vi "LowIF_audiojack_exe_beep.vi"() -> ()   [LabVIEW 2015]
doc: "This example demonstrates how to use the Short-time Fourier Transform (STFT Spectrograms) VI to analyze the Time-Frequency spectrogram."
uses:
  <vilib>/sound2/lvsound2.llb/Sampling Mode.ctl
  <vilib>/Analysis/3filter.llb/Filter Passband Type.ctl
  <vilib>/Analysis/2dsp.llb/Complex FFT.vi
  <vilib>/sound2/lvsound2.llb/Sound Input Read (DBL).vi
  <vilib>/Analysis/3filter.llb/Chebyshev Filter (DBL).vi
  <vilib>/Analysis/baseanly.llb/Mean (CDB).vi
  HeartRate_Global.vi
  <vilib>/Analysis/NI_AALPro.lvlib
  <vilib>/Analysis/NI_AALBase.lvlib
  <vilib>/Analysis/NI_AAL_SigProc.lvlib
panel:
  in  "Data path":path=path "test.lvm" caption="Filename"
  in  "Save":bool=TRUE caption="Enable"
  in  "Beep?":bool=TRUE
  out "Heart rate":dbl format="%#.0f"
  out "Respiration rate":dbl format="%#.0f"
  in  "Minimun dB":dbl=-15.0 max=0.0
  in  "Frequency Range":dbl(slide)=3.2 caption="Beats per Min (x60)" min=1.0 step=0.1 scale=0.0..160.0
  out "Frequency":dbl[](graph) caption="I/Q Signal"
  in  "bits per sample":i32=16
  in  "number of channels":i32=2
  in  "sample rate (S/s)":dbl=320.0
  in  "data length":i32=4800
  out "I/Q Signal":dynamicdata(graph)
  in  "number of samples/ch":i32=32
  in  "device ID":u32
  in  "Stop":bool
  # "Low-IF interferometry radar data processing"
  # "Version: 3\nZhengyu Peng\nC. Li Lab\nTexas Tech University\nOct. 2015"
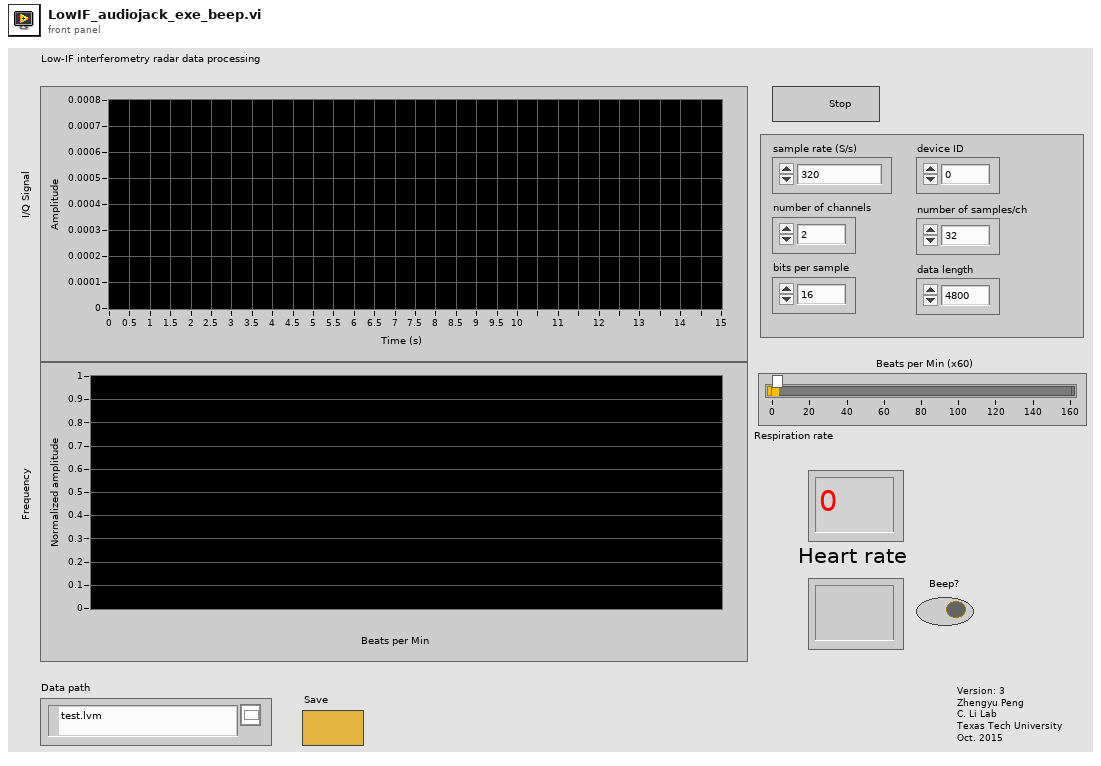
[diagram p1: front panel]
types:
  T1 = typedef "Sampling Mode.ctl" = i32
  T2 = cluster{"sample rate (S/s)":dbl, "number of channels":i32, "bits per sample ":i32}
  T3 = typedef "Sound Input Task ID.ctl" = u32
  T4 = typedef "NI_AALBase.lvlib/Filter Passband Type.ctl" = enum32{"Lowpass", "Highpass", "Bandpass", "Bandstop"}
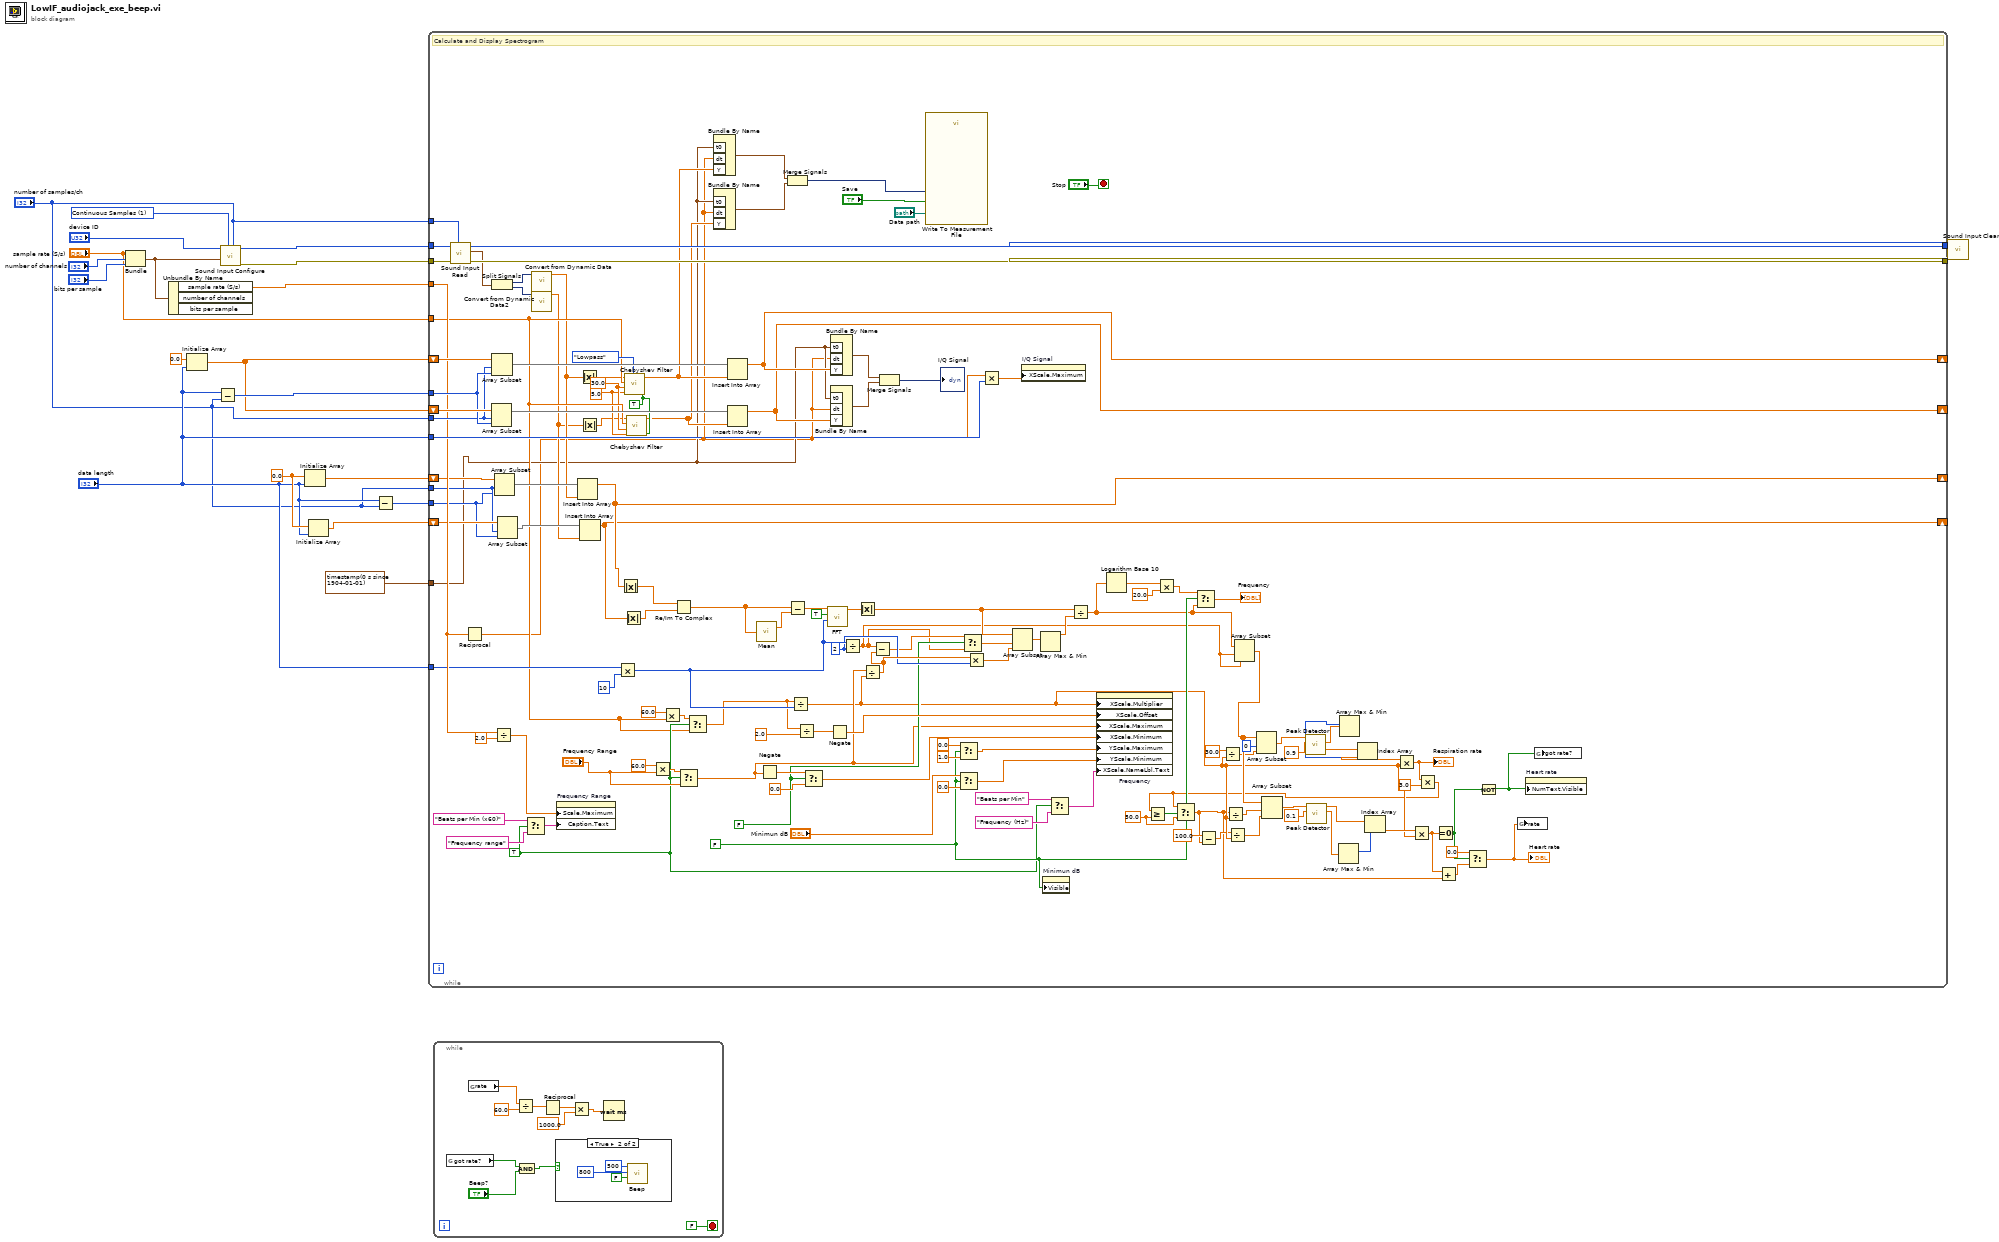
[diagram p0: block diagram]
diagram:
  w4 = T1 1 items=["Finite Samples", "Continuous Samples"] ("sample mode")
  w9 = 0.0 ("element")
  n1 = Bundle("sample rate (S/s)"="sample rate (S/s)", "number of channels"="number of channels", "bits per sample"="bits per sample") -> (w5:T2)  [unwired: 1 in]
  n2 = Unbundle By Name(w5) -> ("sample rate (S/s)"=w13:dbl)  [unwired: 2 out]
  n3 = Initialize Array(0.0 ("element"), "data length") -> (w14:dbl[])
  n4 = Subtract(x="data length", y="number of samples/ch") -> (x-y=w15:i32)
  n5 = call <vilib>:"Sound Input Configure.vi"("number of samples/ch"="number of samples/ch", "sample mode"=w4, "sound format"=w5, "device ID"="device ID") -> ("error out"=w19:errorcluster, "task ID"=w20:T3)  [unwired: 6 in]
  n6 = Initialize Array(w9, "data length") -> (w11:dbl[])
  n7 = Initialize Array(w9, "data length") -> (w8:dbl[])
  n8 = Subtract(x="data length", y="number of samples/ch") -> (x-y=w10:i32)
  n9 = while {
    tunnel: w20 -> [w156]
    tunnel: "number of samples/ch" -> [w155]
    tunnel: w19 -> [w154]
    tunnel: [w153] -> w18
    tunnel: [w152] -> w17
    shift-right: [w137] -> _
    shift-left: w14 -> [w149]
    tunnel: w15 -> [w146]
    shift-right: [w136] -> _
    shift-left: w14 -> [w147]
    tunnel: "number of samples/ch" -> [w143]
    tunnel: w13 -> [w139]
    tunnel: "data length" -> [w141]
    tunnel: "data length" -> [w123]
    tunnel: "sample rate (S/s)" -> [w64]
    shift-right: [w81] -> _
    shift-left: w11 -> [w129]
    tunnel: w10 -> [w125]
    tunnel: "number of samples/ch" -> [w126]
    shift-right: [w79] -> _
    shift-left: w8 -> [w127]
    tunnel: timestamp(0 s since 1904-01-01) ("t0") -> [w28]
    stop <- "Stop" stop-if-true
    w39 = 50.0 ("y")
    w63 = 30.0 ("high cutoff freq: fh")
    w61 = TRUE ("init/cont (init:F)")
    w62 = 5.0 ("high cutoff freq: fh")
    w107 = FALSE ("negative frequency?")
    w97 = FALSE ("dB scale?")
    w84 = TRUE ("scale to beats per min?")
    w110 = 2 ("y")
    # "Calculate and Display Spectrogram"
    n10 = call-poly <vilib>:"Sound Input Read.vi"("number of samples/ch"=w155, "error in (no error)"=w154, "task ID"=w156) -> ("error out"=w152:errorcluster, "data"=w33:waveform(dbl)[], "task ID out"=w153:T3)  [unwired: 6 in]
    n11 = Reciprocal(x=w139) -> (1/x=w27:dbl)
    n12 = Array Subset(array=w147, index=w143, length=w146) -> (w145:dbl[])
    n13 = Split Signals(w33) -> (w151:dynamicdata, w150:dynamicdata)  [unwired: 2 out]
    n14 = Array Subset(array=w149, index=w143, length=w146) -> (w148:dbl[])
    n15 = Divide(x=w139, y=2.0) -> (x/y=w120:dbl)
    n16 = Array Subset(array=w129, index=w126, length=w125) -> (w128:dbl[])
    n17 = Array Subset(array=w127, index=w126, length=w125) -> (w124:dbl[])
    n18 = Select(t="Beats per Min (x60)" ("X Scale.Name Label.Text"), s=w84, f="Frequency range" ("X Scale.Name Label.Text")) -> (s? t:f=w83:string)
    n19 = call "Convert from Dynamic Data"("Dynamic Data Type"=w151) -> ("Array"=w36:dbl[])  [unwired: 3 out]
    n20 = call "Convert from Dynamic Data2"("Dynamic Data Type"=w150) -> ("Array"=w35:dbl[])  [unwired: 3 out]
    n21 = property on="Frequency Range" class="Slide (strict)"("Scale.Maximum"=w120, "Caption.Text"=w83) -> ()  [unwired: 2 in, 2 out]
    n22 = Insert Into Array(array=w128, new element=w36) -> (w81:dbl[])  [unwired: 1 in]
    n23 = Absolute Value(x=w36) -> (abs(x)=w38:dbl[])
    n24 = Absolute Value(x=w35) -> (abs(x)=w37:dbl[])
    n25 = Insert Into Array(array=w124, new element=w35) -> (w79:dbl[])  [unwired: 1 in]
    n26 = Multiply(x=w123, y=10) -> (x*y=w113:i32)
    n27 = Absolute Value(x=w81) -> (abs(x)=w80:dbl[])
    n28 = Absolute Value(x=w79) -> (abs(x)=w78:dbl[])
    n29 = call-poly <vilib>:"Chebyshev Filter.vi"("init/cont (init:F)"=w61, "filter type"=Filter_Passband_Type."Lowpass", "low cutoff freq: fl"=w62, "high cutoff freq: fh"=w63, "sampling freq: fs"=w64, "X"=w38) -> ("Filtered X"=w30:dbl[])  [unwired: 4 in, 1 out]
    n30 = call-poly <vilib>:"Chebyshev Filter.vi"("init/cont (init:F)"=w61, "low cutoff freq: fl"=w62, "high cutoff freq: fh"=w63, "sampling freq: fs"=w64, "X"=w37) -> ("Filtered X"=w29:dbl[])  [unwired: 5 in, 1 out]
    n31 = Multiply(x=60.0, y="Frequency Range") -> (x*y=w89:dbl)
    n32 = Multiply(x=60.0, y=w64) -> (x*y=w92:dbl)
    n33 = Re/Im To Complex(1:w78, 2:w80) -> (0:w82:cdb[])
    n34 = Select(t=w89, s=w84, f="Frequency Range") -> (s? t:f=w88:dbl)
    n35 = Select(t=w92, s=w84, f=w64) -> (s? t:f=w91:dbl)
    n36 = Bundle By Name("t0"=w28, "dt"=w27, "Y"=w30) -> (w26:waveform(dbl))  [unwired: 1 out]
    n37 = Bundle By Name("t0"=w28, "dt"=w27, "Y"=w29) -> (w25:waveform(dbl))  [unwired: 1 out]
    n38 = Insert Into Array(array=w148, new element=w30) -> (w137:dbl[])  [unwired: 1 in]
    n39 = Insert Into Array(array=w145, new element=w29) -> (w136:dbl[])  [unwired: 1 in]
    n40 = call-poly <vilib>:"Mean.vi"("X"=w82) -> ("mean"=w135:cdb)  [unwired: 1 out]
    n41 = Negate(x=w88) -> (-x=w117:dbl)
    n42 = Merge Signals(w26, w25) -> (w24:dynamicdata)
    n43 = Subtract(x=w82, y=w135) -> (x-y=w121:cdb[])
    n44 = Divide(x=w91, y=w113) -> (x/y=w50:dbl)
    n45 = Divide(x=w91, y=2.0) -> (x/y=w131:dbl)
    n46 = Select(t=w117, s=w107, f=0.0) -> (s? t:f=w119:dbl)
    n47 = call-poly <vilib>:"FFT.vi"("FFT size"=w113, "shift?"=TRUE, "X"=w121) -> ("FFT {X}"=w133:cdb[])  [unwired: 7 in, 1 out]
    n48 = Negate(x=w131) -> (-x=w130:dbl)
    n49 = Bundle By Name("t0"=w28, "dt"=w27, "Y"=w137) -> (w144:waveform(dbl))  [unwired: 1 out]
    n50 = Bundle By Name("t0"=w28, "dt"=w27, "Y"=w136) -> (w142:waveform(dbl))  [unwired: 1 out]
    n51 = Divide(x=w113, y=w110) -> (x/y=w47:dbl)
    n52 = Absolute Value(x=w133) -> (abs(x)=w116:dbl[])
    n53 = Divide(x=w88, y=w50) -> (x/y=w111:dbl)
    n54 = Subtract(x=w47, y=w111) -> (x-y=w108:dbl)
    n55 = Merge Signals(w144, w142) -> (→"I/Q Signal":dynamicdata)
    n56 = call "Write To Measurement File"("Signals"=w24, "Enable"="Save", "Filename"="Data path") -> ()  [unwired: 14 in, 3 out]
    n57 = Select(t=0.0, s=w97, f=1.0) -> (s? t:f=w99:dbl)
    n58 = Select(t="Minimun dB", s=w97, f=0.0) -> (s? t:f=w103:dbl)
    n59 = Select(t=w108, s=w107, f=w47) -> (s? t:f=w109:dbl)
    n60 = Multiply(x=w111, y=w110) -> (x*y=w112:dbl)
    n61 = Multiply(x=w27, y=w141) -> (x*y=w140:dbl)
    n62 = Array Subset(array=w116, index=w109, length=w112) -> (w115:dbl[])
    n63 = property on="I/Q Signal" class="WFGraph (strict)"("XScale.Maximum"=w140) -> ()  [unwired: 2 in, 2 out]
    n64 = Array Max & Min(array=w115) -> (max value=w114:dbl)  [unwired: 3 out]
    n65 = property on="Minimun dB" class="DigNum (strict)"("Visible"=w97) -> ()  [unwired: 2 in, 2 out]
    n66 = Select(t="Beats per Min" ("X Scale.Name Label.Text"), s=w84, f="Frequency (Hz)" ("X Scale.Name Label.Text")) -> (s? t:f=w95:string)
    n67 = Divide(x=w116, y=w114) -> (x/y=w68:dbl[])
    n68 = property on="Frequency" class="WFGraph (strict)"("XScale.Multiplier"=w50, "XScale.Offset"=w130, "XScale.Maximum"=w88, "XScale.Minimum"=w119, "YScale.Maximum"=w99, "YScale.Minimum"=w103, "XScale.NameLbl.Text"=w95) -> ()  [unwired: 2 in, 2 out]
    n69 = Logarithm Base 10(1:w68) -> (0:w106:dbl[])
    n70 = Multiply(x=w106, y=20.0) -> (x*y=w76:dbl[])
    n71 = Select(t=w76, s=w97, f=w68) -> (s? t:f=→"Frequency":dbl[])
    n72 = Divide(x=30.0, y=w50) -> (x/y=w52:dbl)
    n73 = Array Subset(array=w68, index=w47, length=w47) -> (w54:dbl[])
    n74 = Array Subset(array=w54, index=0, length=w52) -> (w55:dbl[])
    n75 = call <vilib>:"Peak Detector.vi"("threshold"=0.9, "X"=w55) -> ("Amplitudes"=w59:dbl[], "Locations"=w60:dbl[])  [unwired: 5 in, 3 out]
    n76 = Array Max & Min(array=w59) -> (max index (indices)=w58:i32)  [unwired: 3 out]
    n77 = Index Array(array=w60, index=w58) -> (element=w75:dbl)
    n78 = Multiply(x=w75, y=w50) -> (x*y=w46:dbl)
    "Respiration rate" <- w46
    n79 = Multiply(x=w46, y=3.0) -> (x*y=w41:dbl)
    n80 = Greater Or Equal?(x=w41, y=w39) -> (x >= y?=w42:bool)
    n81 = Select(t=w41, s=w42, f=w39) -> (s? t:f=w40:dbl)
    n82 = Subtract(x=100.0, y=w40) -> (x-y=w43:dbl)
    n83 = Divide(x=w40, y=w50) -> (x/y=w74:dbl)
    n84 = Divide(x=w43, y=w50) -> (x/y=w73:dbl)
    n85 = Array Subset(array=w54, index=w74, length=w73) -> (w72:dbl[])
    n86 = call <vilib>:"Peak Detector.vi"("threshold"=0.1, "X"=w72) -> ("Amplitudes"=w57:dbl[], "Locations"=w70:dbl[])  [unwired: 5 in, 3 out]
    n87 = Array Max & Min(array=w57) -> (max index (indices)=w56:i32)  [unwired: 3 out]
    n88 = Index Array(array=w70, index=w56) -> (element=w69:dbl)
    n89 = Multiply(x=w69, y=w50) -> (x*y=w66:dbl)
    n90 = Equal To 0?(x=w66) -> (x = 0?=w48:bool)
    n91 = Add(x=w66, y=w40) -> (x+y=w67:dbl)
    n92 = Select(t=0.0, s=w48, f=w67) -> (s? t:f=w32:dbl)
    "Heart rate" <- w32
    n93 = Not(x=w48) -> (.not. x?=w31:bool)
    n94 = global write "HeartRate_Global.vi" "rate"(w32) -> ()
    n95 = property on="Heart rate" class="DigNum (strict)"("NumText.Visible"=w31) -> ()  [unwired: 2 in, 2 out]
    n96 = global write "HeartRate_Global.vi" "got rate?"(w31) -> ()
  }
  n97 = while {
    stop <- FALSE stop-if-true
    n98 = global read "HeartRate_Global.vi" "got rate?"() -> (w159:bool)
    n99 = global read "HeartRate_Global.vi" "rate"() -> (w161:dbl)
    n100 = Divide(x=w161, y=60.0) -> (x/y=w165:dbl)
    n101 = And(x=w159, y="Beep?") -> (x .and. y?=w158:bool)
    n102 = Reciprocal(x=w165) -> (1/x=w164:dbl)
    n103 = case shown="True" w158 {
      frame False {
      }
      frame True {
        n104 = call <vilib>:"Beep.vi"("use system alert? (T)"=FALSE, "duration (msec)"=u32 800, "frequency (Hz)"=u32 500) -> ()  [unwired: 9 in]
      }
    }
    n105 = Multiply(x=w164, y=1000.0) -> (x*y=w162:dbl)
    n106 = Wait (ms)(milliseconds to wait=w162) -> ()  [unwired: 1 out]
  }
  n107 = call <vilib>:"Sound Input Clear.vi"("error in (no error)"=w17, "task ID"=w18) -> ()  [unwired: 9 in, 1 out]
